vi "ValueSignalByPathString.vi"(0 "VI Reference In":refnum<vi>, 2 "delimiter (>>)":string=">>", 5 "Control Name":string, 7 "Value (Signaling)":variant, 11 "error in":errorcluster) -> (4 "VI Reference Out":refnum<vi>, 15 "error out":errorcluster)   [LabVIEW 2016, in "Drona.lvlib" / "ValueSignal.lvlib"]
doc: "Sets the value of controls. \nThe input control name is given as a string , incase of path, use delimiters inbetween the path."
uses:
  ValueSignal.lvlib
  Drona.lvlib
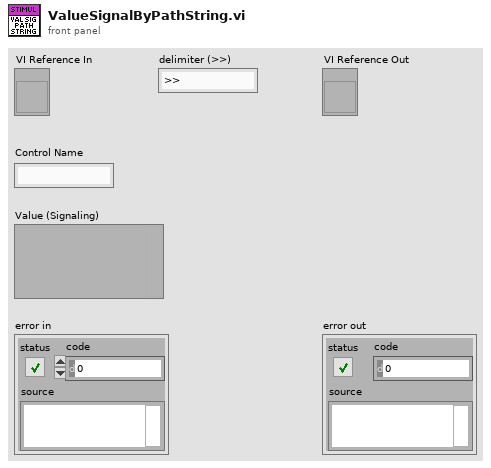
[diagram p1: front panel]
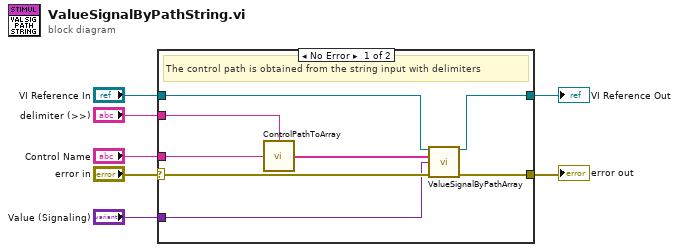
[diagram p0: block diagram]
diagram:
  n1 = case shown="No Error" "error in" {
    selector: "error in" -> [w15 w17]
    tunnel: "Control Name" -> [w10 _]
    tunnel: "VI Reference In" -> [w12 w16]
    tunnel: [w11 w16] -> w4
    tunnel: "Value (Signaling)" -> [w13 _]
    tunnel: [w14 w17] -> w2
    tunnel: "delimiter (>>)" -> [w8 _]
    frame No Error {
      # "The control path is obtained from the string input with delimiters"
      n2 = call "ControlPathToArray.vi"("Control Name"=w10, "delimiter (>>)"=w8) -> ("Control Path"=w9:string[])
      n3 = call "ValueSignalByPathArray.vi"("VI Reference In"=w12, "Control Path"=w9, "Value (Signaling)"=w13, "error in"=w15) -> ("VI Reference Out"=w11:refnum<vi>, "error out"=w14:errorcluster)  [unwired: 10 in]
    }
    frame Error {
    }
  }
  "error out" <- w2
  "VI Reference Out" <- w4
